vi "equipment_debug.vi"() -> ()   [LabVIEW 2017]
uses:
  <vilib>/Instr/_visa.llb/VISA Configure Serial Port (Instr).vi
panel:
  out "控制板正常？":bool
  in  "控制板":refnum<visa-resource-name>
  in  "退出":bool
  in  "连通性测试":bool
  out "DH1766-2正常？":bool
  out "HP34401正常?":bool
  out "CONST820正常?":bool
  out "GWS正常？":bool
  in  "DH1766-2":refnum<visa-resource-name>
  in  "HP34401":refnum<visa-resource-name>
  in  "CONST820":refnum<visa-resource-name>
  in  "GWS":refnum<visa-resource-name>
  # "设备通信检查"
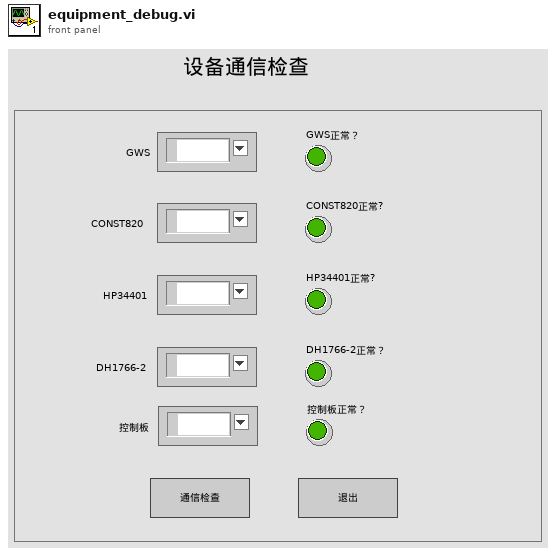
[diagram p1: front panel]
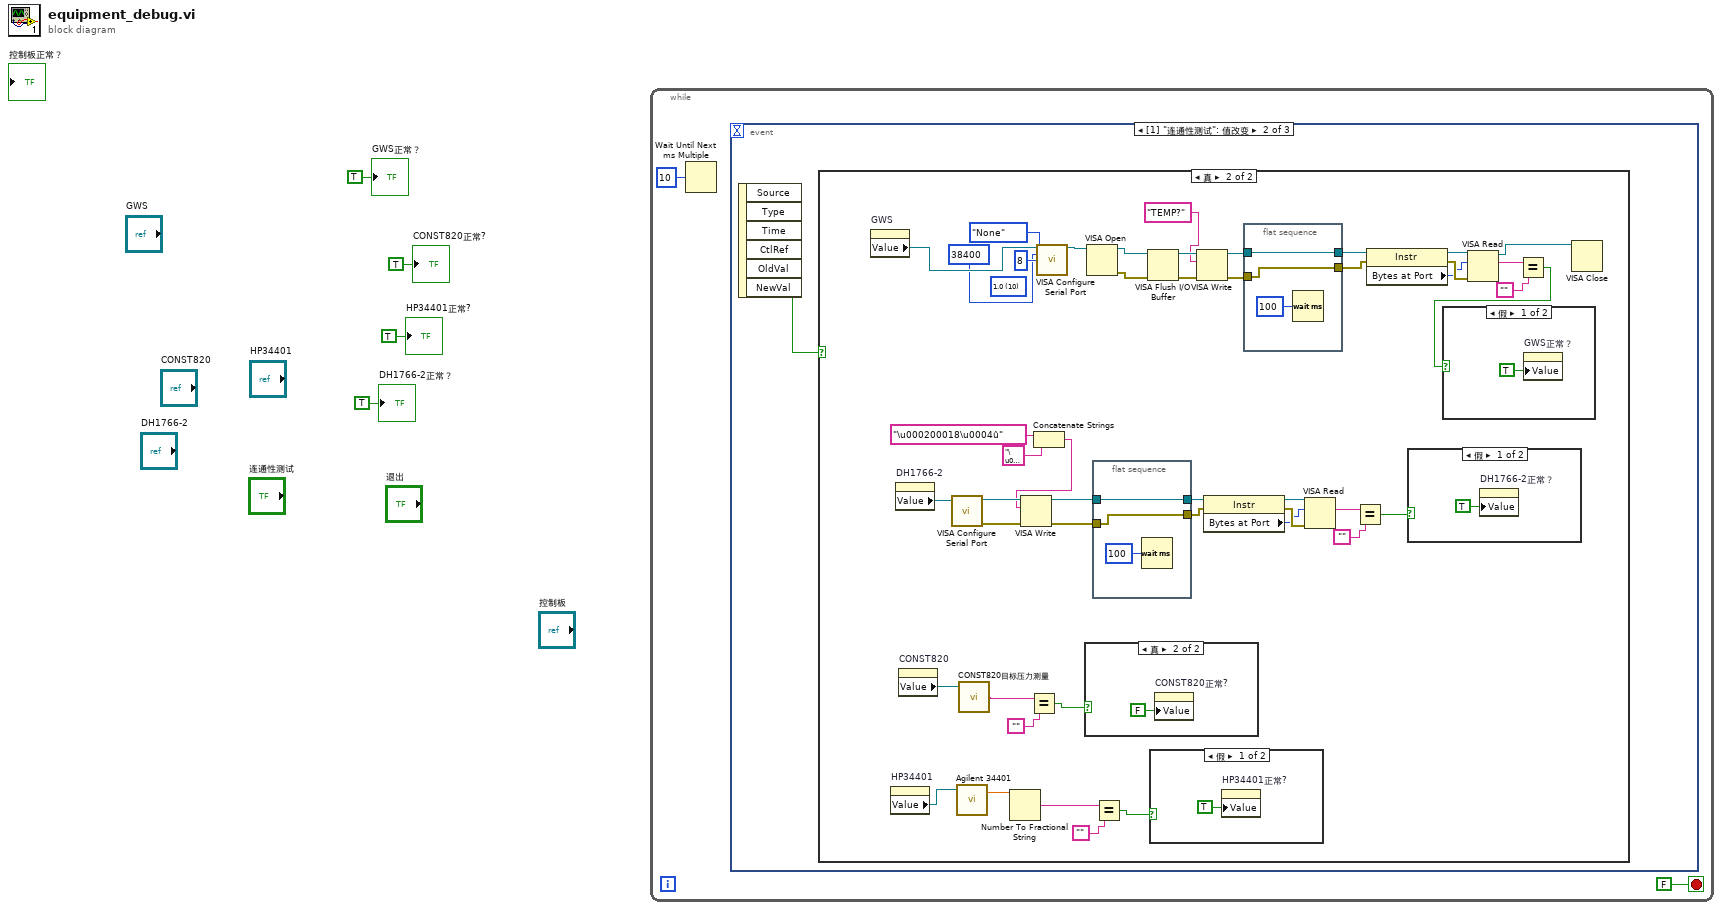
[diagram p0: block diagram]
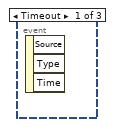
[diagram p2: hidden frame]
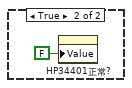
[diagram p4: hidden frame]
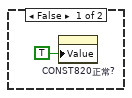
[diagram p5: hidden frame]
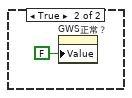
[diagram p6: hidden frame]
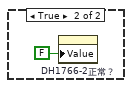
[diagram p7: hidden frame]
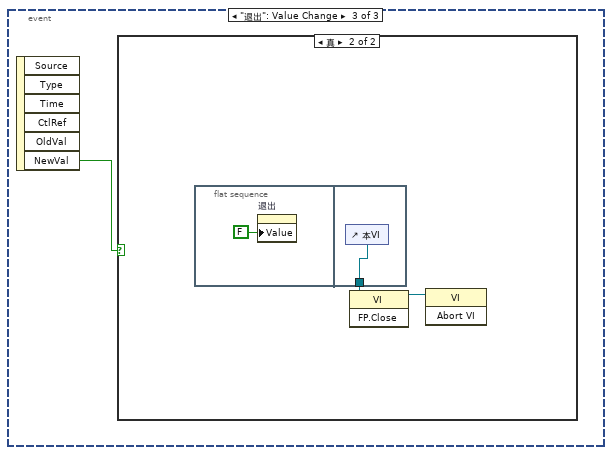
[diagram p8: hidden frame]
diagram:
  n1 = while {
    stop <- FALSE stop-if-true
    n2 = Wait Until Next ms Multiple(millisecond multiple=u32 10 ("毫秒倍数")) -> ()  [unwired: 1 out]
    n3 = event shown="[1] \"连通性测试\": 值改变" {
      selector: _ -> [_ _ _]
      dyn-events: _ -> [_ _ _]
      timeout: _ -> [_ _ _]
      event Timeout {
        n4 = event-data() -> ()  [unwired: 1 in, 3 out]
      }
      event "连通性测试": Value Change {
        n5 = event-data() -> ("NewVal"=w7:bool)  [unwired: 1 in, 5 out]
        n6 = case shown="真" w7 {
          frame False {
          }
          frame True {
            (unwired) u16 10 items=["1.0"=10, "1.5"=15, "2.0"=20] ("stop bits (10: 1 bit)")
            n7 = property on="GWS" class="VISAName"() -> ("Value"=w50:refnum<visa-resource-name>)  [unwired: 2 in, 2 out]
            n8 = property on="HP34401" class="VISAName"() -> ("Value"=w13:refnum<visa-resource-name>)  [unwired: 2 in, 2 out]
            n9 = property on="DH1766-2" class="VISAName"() -> ("Value"=w48:refnum<visa-resource-name>)  [unwired: 2 in, 2 out]
            n10 = property on="CONST820" class="VISAName"() -> ("Value"=w17:refnum<visa-resource-name>)  [unwired: 2 in, 2 out]
            n11 = call-poly "VISA Configure Serial Port"("VISA resource name"=w48) -> ("VISA resource name out"=w45:refnum<visa-resource-name>, "error out"=w43:errorcluster)  [unwired: 13 in]
            n12 = call "Agilent 34401.vi"("VISA resource name"=w13) -> ("Measurement"=w12:dbl)  [unwired: 2 in, 1 out]
            n13 = call "CONST820目标压力测量.vi"("VISA resource name"=w17) -> ("目标压力值"=w15:string)  [unwired: 2 in, 2 out]
            n14 = Number To Fractional String(number=w12) -> (F-format string=w9:string)  [unwired: 3 in]
            n15 = Equal?(x=w15, y="") -> (x = y?=w14:bool)
            n16 = Concatenate Strings("\u000200018\u0004û" ("字符串"), "\u0003" ("字符串")) -> (w44:string)
            n17 = VISA Write(VISA resource name=w45, write buffer=w44, error in (no error)=w43) -> (VISA resource name out=w42:refnum<visa-resource-name>, error out=w40:errorcluster)  [unwired: 1 out]
            n18 = call-poly "VISA Configure Serial Port"("VISA resource name"=w50, "baud rate (9600)"=u32 38400, "data bits (8)"=u16 8, "parity (0:none)"=enum16{"None", "Odd", "Even", "Mark", "Space"}."None") -> ("VISA resource name out"=w53:refnum<visa-resource-name>)  [unwired: 10 in, 1 out]
            n19 = case shown="真" w14 {
              frame False {
                n20 = property on="CONST820正常?" class="Bool (严格)"("Value"=TRUE ("DH1766-2正常？")) -> ()  [unwired: 2 in, 2 out]
              }
              frame True {
                n21 = property on="CONST820正常?" class="Bool (严格)"("Value"=FALSE ("DH1766-2正常？")) -> ()  [unwired: 2 in, 2 out]
              }
            }
            n22 = VISA Open(VISA resource name=w53) -> (VISA resource name=w29:refnum<visa-resource-name>, error out=w28:errorcluster)  [unwired: 4 in]
            n23 = flat-sequence {
              tunnel: w42 -> [w66]
              tunnel: [w66] -> w41
              tunnel: w40 -> [w65]
              tunnel: [w65] -> w39
              frame #0 {
                n24 = Wait (ms)(milliseconds to wait=u32 100 ("等待时间（毫秒）")) -> ()  [unwired: 1 out]
              }
            }
            n25 = Equal?(x=w9, y="") -> (x = y?=w10:bool)
            n26 = VISA Flush I/O Buffer(VISA resource name=w29, error in (no error)=w28) -> (VISA resource name out=w31:refnum<visa-resource-name>, error out=w32:errorcluster)  [unwired: 1 in]
            n27 = case shown="假" w10 {
              frame False {
                n28 = property on="HP34401正常?" class="Bool (严格)"("Value"=TRUE ("DH1766-2正常？")) -> ()  [unwired: 2 in, 2 out]
              }
              frame True {
                n29 = property on="HP34401正常?" class="Bool (严格)"("Value"=FALSE ("DH1766-2正常？")) -> ()  [unwired: 2 in, 2 out]
              }
            }
            n30 = VISA Write(VISA resource name=w31, write buffer="TEMP?" ("写入缓冲区"), error in (no error)=w32) -> (VISA resource name out=w27:refnum<visa-resource-name>, error out=w26:errorcluster)  [unwired: 1 out]
            n31 = property class="Instr"(reference=w41, error in=w39) -> (reference out=w36:refnum<visa-resource-name>, error out=w38:errorcluster, "Bytes at Port"=w37:u32)
            n32 = flat-sequence {
              tunnel: w27 -> [w61]
              tunnel: [w61] -> w20
              tunnel: w26 -> [w60]
              tunnel: [w60] -> w19
              frame #0 {
                n33 = Wait (ms)(milliseconds to wait=u32 100 ("等待时间（毫秒）")) -> ()  [unwired: 1 out]
              }
            }
            n34 = VISA Read(VISA resource name=w36, byte count=w37, error in (no error)=w38) -> (read buffer=w35:string)  [unwired: 3 out]
            n35 = Equal?(x=w35, y="") -> (x = y?=w33:bool)
            n36 = property class="Instr"(reference=w20, error in=w19) -> (reference out=w23:refnum<visa-resource-name>, error out=w25:errorcluster, "Bytes at Port"=w24:u32)
            n37 = case shown="假" w33 {
              frame False {
                n38 = property on="DH1766-2正常？" class="Bool (严格)"("Value"=TRUE ("DH1766-2正常？")) -> ()  [unwired: 2 in, 2 out]
              }
              frame True {
                n39 = property on="DH1766-2正常？" class="Bool (严格)"("Value"=FALSE ("DH1766-2正常？")) -> ()  [unwired: 2 in, 2 out]
              }
            }
            n40 = VISA Read(VISA resource name=w23, byte count=w24, error in (no error)=w25) -> (VISA resource name out=w8:refnum<visa-resource-name>, read buffer=w22:string)  [unwired: 2 out]
            n41 = Equal?(x=w22, y="") -> (x = y?=w18:bool)
            n42 = case shown="假" w18 {
              frame False {
                n43 = property on="GWS正常？" class="Bool (严格)"("Value"=TRUE ("GWS正常？")) -> ()  [unwired: 2 in, 2 out]
              }
              frame True {
                n44 = property on="GWS正常？" class="Bool (严格)"("Value"=FALSE ("GWS正常？")) -> ()  [unwired: 2 in, 2 out]
              }
            }
            n45 = VISA Close(VISA resource name=w8) -> ()  [unwired: 1 in, 1 out]
          }
        }
      }
      event "退出": Value Change {
        n46 = event-data() -> ("NewVal"=w68:bool)  [unwired: 1 in, 5 out]
        n47 = case shown="真" w68 {
          frame False {
          }
          frame True {
            n48 = flat-sequence {
              tunnel: [w72] -> w70
              frame #0 {
                n49 = property on="退出" class="Bool (严格)"("Value"=FALSE ("退出")) -> ()  [unwired: 2 in, 2 out]
              }
              frame #1 {
                n50 = control-ref of="本VI"() -> (w72:refnum<vi>)
              }
            }
            n51 = invoke class="VI" method="FP.Close"(reference=w70) -> (reference out=w69:refnum<vi>)  [unwired: 2 in, 2 out]
            n52 = invoke class="VI" method="Abort VI"(reference=w69) -> ()  [unwired: 2 in, 3 out]
          }
        }
      }
    }
  }
  "GWS正常？" <- TRUE ("GWS正常？")
  "CONST820正常?" <- TRUE ("CONST820正常?")
  "HP34401正常?" <- TRUE ("HP34401正常?")
  "DH1766-2正常？" <- TRUE ("DH1766-2正常？")
